vi "01 - PXI Modular Instruments.vi"   [LabVIEW 2021]
uses:
  <resource>/objmgr/RFmxSpecAn.rc
  <instrlib>/niSwitch/niSwitch.llb/niSwitch Connect Channels (Multiple).vi
  <vilib>/RFmx/SpecAn/mx/RFmxSpecAn.llb/RFmxSpecAn Spectrum Fetch Measurement.vi
  <instrlib>/niScope/Acquire/Fetch/niScope Fetch Cluster.vi
panel:
  # "Open Block Diagram to see PXI Hardware Connections\nCtl + E (instructions on diagram)"
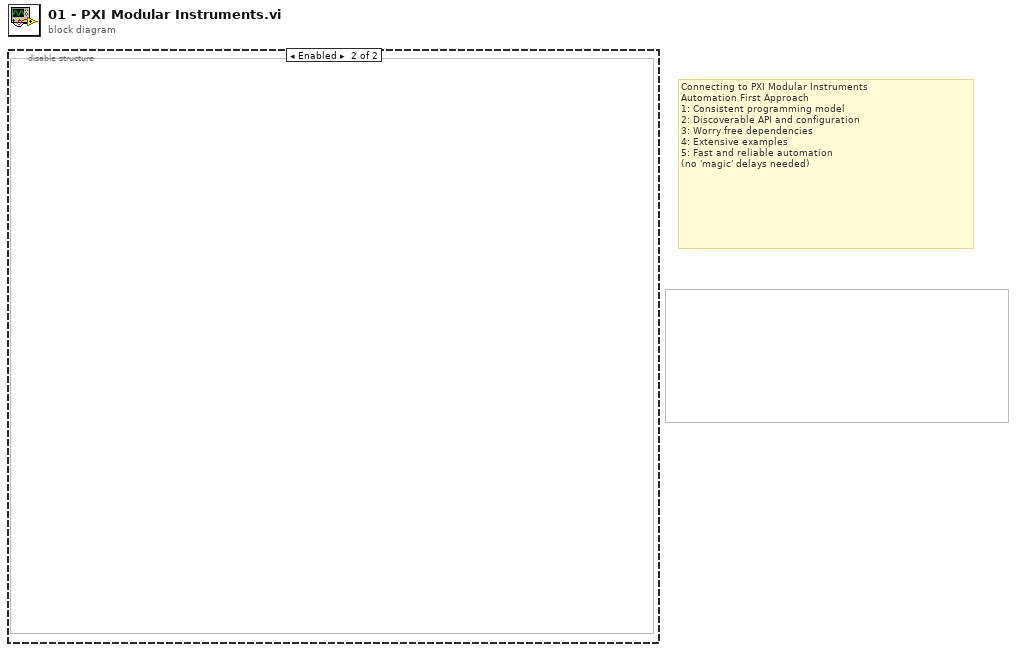
[diagram p0: block diagram]
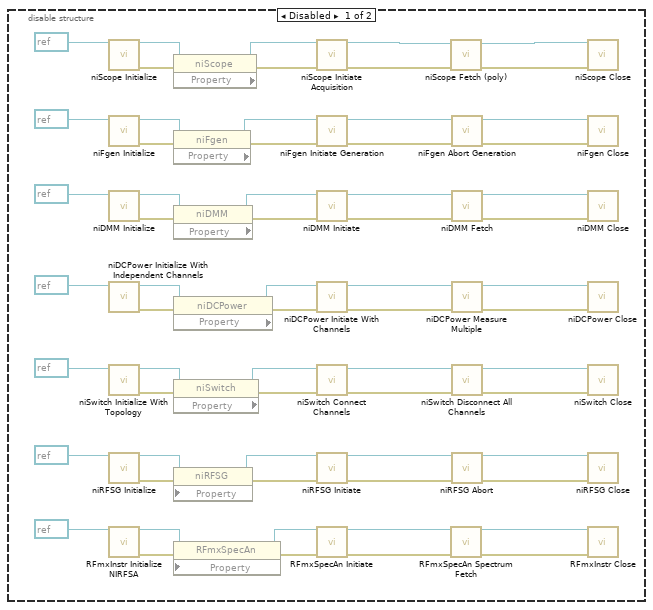
[diagram p2: hidden frame]
diagram:
  # "Connecting to PXI Modular Instruments\nAutomation First Approach\n1: Consistent programming model\n2: Discoverable API and configuration\n3: Worry free dependencies\n4: Extensive examples\n5: Fast and reliable automation\n(no 'magic' delays needed)"
  n1 = disable-structure shown="Enabled" {
    frame Disabled {
      n2 = call <instrlib>:"niScope Initialize.vi"("resource name"=refnum<k15> refnum) -> ("instrument handle"=w21:refnum<k15>, "error out"=w63:errorcluster)  [unwired: 13 in]
      n3 = call <instrlib>:"niFgen Initialize.vi"("Resource Name"=refnum<k15> refnum) -> ("error out"=w57:errorcluster, "Instrument Handle Out"=w20:refnum<k15>)  [unwired: 9 in]
      n4 = call <instrlib>:"niDMM Initialize.vi"("Instrument Descriptor"=refnum<k15> refnum) -> ("error out"=w49:errorcluster, "instrument handle out"=w19:refnum<k15>)  [unwired: 9 in]
      n5 = call <instrlib>:"niDCPower Initialize With Independent Channels.vi"("resource name"=refnum<k15> refnum) -> ("error out"=w44:errorcluster, "instrument handle out"=w18:refnum<k15>)  [unwired: 9 in]
      n6 = call <instrlib>:"niSwitch Initialize With Topology.vi"("resource name"=refnum<k15> refnum) -> ("error out"=w39:errorcluster, "instrument handle out"=w17:refnum<k15>)  [unwired: 9 in]
      n7 = call <instrlib>:"niRFSG Initialize.vi"("resource name"=refnum<k15> refnum) -> ("instrument handle"=w16:refnum<k15>, "error out"=w32:errorcluster)  [unwired: 13 in]
      n8 = call <vilib>:"RFmxInstr Initialize NIRFSA.vi"("Resource Name"=refnum<k15> refnum) -> ("Instrument Handle Out"=w15:refnum<k21>, "error out"=w27:errorcluster)  [unwired: 12 in, 1 out]
      n9 = property class="niScope" props=[](reference=w21, error in=w63) -> (reference out=w14:refnum<k15>, error out=w62:errorcluster)  [unwired: 1 out]
      n10 = property class="niFgen" props=[](reference=w20, error in=w57) -> (reference out=w13:refnum<k15>, error out=w56:errorcluster)  [unwired: 1 out]
      n11 = property class="niDMM" props=[](reference=w19, error in=w49) -> (reference out=w12:refnum<k15>, error out=w48:errorcluster)  [unwired: 1 out]
      n12 = property class="niDCPower" props=[](reference=w18, error in=w44) -> (reference out=w11:refnum<k15>, error out=w45:errorcluster)  [unwired: 1 out]
      n13 = property class="niSwitch" props=[](reference=w17, error in=w39) -> (reference out=w10:refnum<k15>, error out=w38:errorcluster)  [unwired: 1 out]
      n14 = property class="niRFSG" props=[](reference=w16, error in=w32) -> (reference out=w9:refnum<k15>, error out=w33:errorcluster)  [unwired: 1 in]
      n15 = property class="RFmxSpecAn" props=[](reference=w15, error in=w27) -> (reference out=w8:refnum<k21>, error out=w26:errorcluster)  [unwired: 1 in]
      n16 = call <instrlib>:"niScope Initiate Acquisition.vi"("instrument handle"=w14, "error in"=w62) -> ("instrument handle out"=w59:refnum<k15>, "error out"=w61:errorcluster)  [unwired: 12 in]
      n17 = call <instrlib>:"niFgen Initiate Generation.vi"("error in (no error)"=w56, "Instrument Handle"=w13) -> ("error out"=w54:errorcluster, "Instrument Handle Out"=w55:refnum<k15>)  [unwired: 8 in]
      n18 = call <instrlib>:"niDMM Initiate.vi"("error in (no error)"=w48, "instrument handle"=w12) -> ("error out"=w46:errorcluster, "instrument handle out"=w47:refnum<k15>)  [unwired: 8 in]
      n19 = call <instrlib>:"niDCPower Initiate With Channels.vi"("error in (no error)"=w45, "instrument handle"=w11) -> ("error out"=w42:errorcluster, "instrument handle out"=w43:refnum<k15>)  [unwired: 8 in]
      n20 = call-poly <instrlib>:"niSwitch Connect Channels.vi"("error in (no error)"=w38, "instrument handle"=w10) -> ("error out"=w36:errorcluster, "instrument handle out"=w37:refnum<k15>)  [unwired: 8 in]
      n21 = call <instrlib>:"niRFSG Initiate.vi"("instrument handle"=w9, "error in"=w33) -> ("instrument handle out"=w31:refnum<k15>, "error out"=w30:errorcluster)  [unwired: 12 in]
      n22 = call <vilib>:"RFmxSpecAn Initiate.vi"("Instrument Handle In"=w8, "error in (no error)"=w26) -> ("Instrument Handle Out"=w25:refnum<k21>, "error out"=w24:errorcluster)  [unwired: 11 in, 1 out]
      n23 = call-poly <instrlib>:"niScope Fetch (poly).vi"("error in"=w61, "instrument handle"=w59) -> ("error out"=w60:errorcluster, "instrument handle out"=w58:refnum<k15>)  [unwired: 6 in, 2 out]
      n24 = call-poly <vilib>:"RFmxSpecAn Spectrum Fetch.vi"("Instrument Handle In"=w25, "error in (no error)"=w24) -> ("Instrument Handle Out"=w23:refnum<k21>, "error out"=w22:errorcluster)  [unwired: 9 in, 3 out]
      n25 = call <instrlib>:"niFgen Abort Generation.vi"("error in (no error)"=w54, "Instrument Handle"=w55) -> ("error out"=w52:errorcluster, "Instrument Handle Out"=w53:refnum<k15>)  [unwired: 8 in]
      n26 = call <instrlib>:"niDMM Fetch.vi"("error in (no error)"=w46, "instrument handle"=w47) -> ("error out"=w51:errorcluster, "instrument handle out"=w50:refnum<k15>)  [unwired: 7 in, 1 out]
      n27 = call <instrlib>:"niDCPower Measure Multiple.vi"("error in (no error)"=w42, "instrument handle"=w43) -> ("error out"=w40:errorcluster, "instrument handle out"=w41:refnum<k15>)  [unwired: 6 in, 2 out]
      n28 = call <instrlib>:"niSwitch Disconnect All Channels.vi"("error in (no error)"=w36, "instrument handle"=w37) -> ("error out"=w34:errorcluster, "instrument handle out"=w35:refnum<k15>)  [unwired: 8 in]
      n29 = call <instrlib>:"niRFSG Abort.vi"("instrument handle"=w31, "error in"=w30) -> ("instrument handle out"=w29:refnum<k15>, "error out"=w28:errorcluster)  [unwired: 12 in]
      n30 = call <instrlib>:"niScope Close.vi"("instrument handle"=w58, "error in"=w60) -> ()  [unwired: 13 in, 1 out]
      n31 = call <instrlib>:"niFgen Close.vi"("error in (no error)"=w52, "Instrument Handle"=w53) -> ()  [unwired: 9 in, 1 out]
      n32 = call <instrlib>:"niDMM Close.vi"("error in (no error)"=w51, "instrument handle"=w50) -> ()  [unwired: 9 in, 1 out]
      n33 = call <instrlib>:"niDCPower Close.vi"("error in (no error)"=w40, "instrument handle"=w41) -> ()  [unwired: 9 in, 1 out]
      n34 = call <instrlib>:"niSwitch Close.vi"("error in (no error)"=w34, "instrument handle"=w35) -> ()  [unwired: 9 in, 1 out]
      n35 = call <instrlib>:"niRFSG Close.vi"("instrument handle"=w29, "error in"=w28) -> ()  [unwired: 13 in, 1 out]
      n36 = call <vilib>:"RFmxInstr Close.vi"("Instrument Handle In"=w23, "error in (no error)"=w22) -> ()  [unwired: 13 in, 1 out]
    }
    frame Enabled {
    }
  }
